vi "Write to DB.vi"(8 "error in":errorcluster, 9 "Chamber ID":T2[](array[typedef])=[{"name"="", "Address"=""}, {"name"="", "Address"=""}], 10 "AML Cluster const":T1[](array[typedef]), 11 "Data.PG in":refnum<class "LV-Data.PGSQL.lvclass">) -> (0 "error out":errorcluster, 2 "Successful Writes":bool[](array[boolean]), 3 "Data.PG out":refnum<class "LV-Data.PGSQL.lvclass">)   [LabVIEW 2019, in "PGC2D.lvlib"]
uses:
  PGC2D.lvlib
  typedefs/Instrument.AML.PGC2D_Chamber_ID--cluster.ctl
  <userlib>/LevyLab/LV-Data/LV-Data.PG/LV-Data.PGSQL.lvclass
  sandbox/Instrument.AML.GetAll--Cluster.ctl
  <userlib>/LevyLab/LV-Data/LV-Data.PG/API/Write Variable (one-row).vi
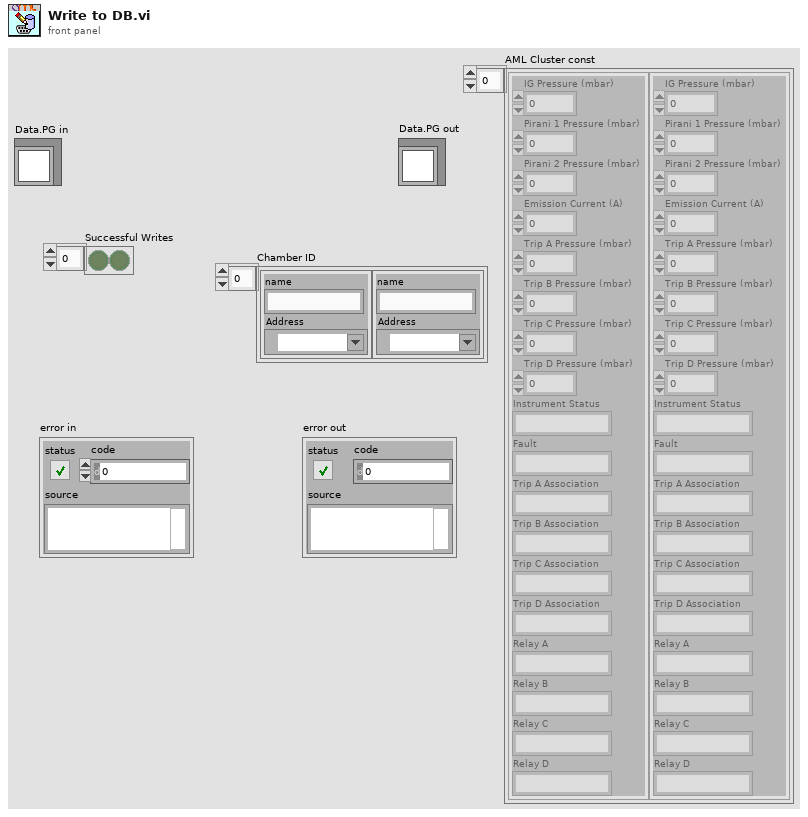
[diagram p1: front panel]
types:
  T1 = typedef "Instrument.AML.GetAll--Cluster.ctl" = cluster{"IG Pressure (mbar)":dbl, "Pirani 1 Pressure (mbar)":dbl, "Pirani 2 Pressure (mbar)":dbl, "Emission Current (A)":dbl, "Trip A Pressure (mbar)":dbl, "Trip B Pressure (mbar)":dbl, "Trip C Pressure (mbar)":dbl, "Trip D Pressure (mbar)":dbl, "Instrument Status":string, "Fault":string, "Trip A Association":string, "Trip B Association":string, "Trip C Association":string, "Trip D Association":string, "Relay A":string, "Relay B":string, "Relay C":string, "Relay D":string}
  T2 = typedef "PGC2D.lvlib/Instrument.AML.PGC2D_Chamber_ID--cluster.ctl" = cluster{"name":string, "Address":refnum<visa-resource-name>}
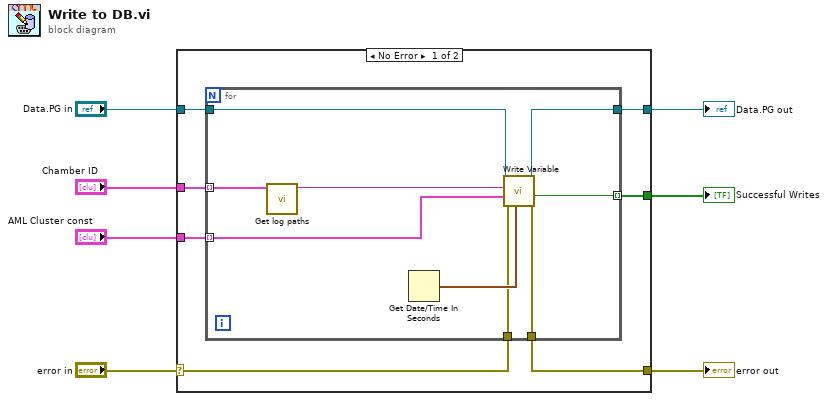
[diagram p0: block diagram]
diagram:
  n1 = case shown="No Error" "error in" {
    selector: "error in" -> [w14 w25]
    tunnel: [w13 w25] -> w6
    tunnel: "Data.PG in" -> [w12 w24]
    tunnel: [w11 w24] -> w4
    tunnel: [w10 _] -> w3
    tunnel: "AML Cluster const" -> [w9 _]
    tunnel: "Chamber ID" -> [w8 _]
    frame No Error {
      n2 = for {
        tunnel: w14 -> [w22]
        tunnel: [w21] -> w13
        tunnel: w12 -> [w20]
        tunnel: [w19] -> w11
        tunnel: [w18] -> w10 mode=indexing
        tunnel: w9 -> [w17] mode=indexing
        tunnel: w8 -> [w15] mode=indexing
        n3 = call "Get log paths.vi"("Chamber ID"=w15) -> ("paths"=w16:string)  [unwired: 10 in]
        n4 = Get Date/Time In Seconds() -> (seconds since 1Jan1904=w23:timestamp)
        n5 = call-poly <userlib>:"Write Variable.vi"("Time Stamp"=w23, "error in (no error)"=w22, "Data"=w17, "variable"=w16, "Data.PG in"=w20) -> ("error out"=w21:errorcluster, "Wrote to DB?"=w18:bool, "Data.PG out"=w19:refnum<class "LV-Data.PGSQL.lvclass">)  [unwired: 3 in, 1 out]
      }
    }
    frame Error {
    }
  }
  "error out" <- w6
  "Data.PG out" <- w4
  "Successful Writes" <- w3
